vi "Lookup Descendants.vi"(7 "Start (Root)":refnum<class "Config Element.lvclass">, 8 "error in (no error)":errorcluster, 10 "Lookup":refnum<class "Config Lookup.lvclass">, 11 "VolatusConfig in":refnum<class "VolatusConfig.lvclass">) -> (0 "error out":errorcluster, 2 "Descendants":refnum<class "Config Element.lvclass">[](array[class]), 3 "VolatusConfig out":refnum<class "VolatusConfig.lvclass">)   [LabVIEW 2020, in "VolatusConfig.lvlib" / "VolatusConfig.lvclass"]
uses:
  VolatusConfig.lvclass
  VolatusConfig.lvclass/VolatusConfig.ctl
  lv-cdm/CDM-Config/Config Manager/Config Manager.lvclass
  lv-cdm/CDM-Config/Config Filter/Config Lookup.lvclass
  lv-cdm/CDM-Config/Config Element/Config Element.lvclass
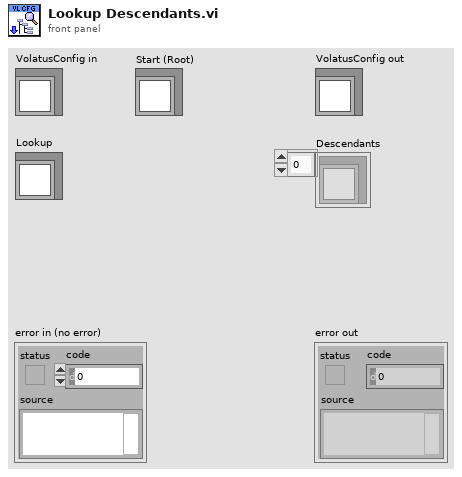
[diagram p1: front panel]
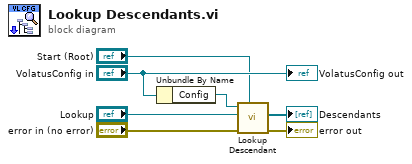
[diagram p0: block diagram]
diagram:
  n1 = Unbundle By Name("VolatusConfig in") -> ("Config"=w6:refnum<class "Config Manager.lvclass">)
  n2 = call "Lookup Descendant.vi"("Start (Root)"="Start (Root)", "error in (no error)"="error in (no error)", "Lookup"="Lookup", "Config Manager in"=w6) -> ("error out"=→"error out":errorcluster, "Descendants"=→"Descendants":refnum<class "Config Element.lvclass">[])  [unwired: 5 in, 1 out]
  "VolatusConfig out" <- "VolatusConfig in"
